vi "Generate Module Definition.vi"(10 "数组":string[][](array[string]), 11 "模块名称":string) -> (3 "模块定义":T1)   [LabVIEW 2018, in "MainInterface.lvlib"]
uses:
  MainInterface.lvlib
  ModuleInterface/ModuleDefinition.ctl
  ModuleInterface/FunctionItem.ctl
  ModuleInterface/ModuleInterface.lvlib
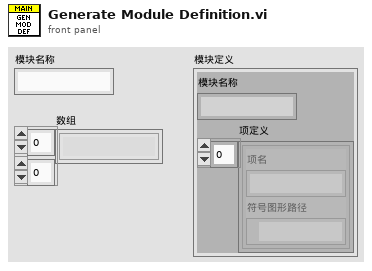
[diagram p1: front panel]
types:
  T1 = typedef "ModuleInterface.lvlib/ModuleDefinition.ctl" = cluster{"模块名称":string, "项定义":T2[]}
  T2 = typedef "ModuleInterface.lvlib/FunctionItem.ctl" = cluster{"项名":string, "符号图形路径":path}
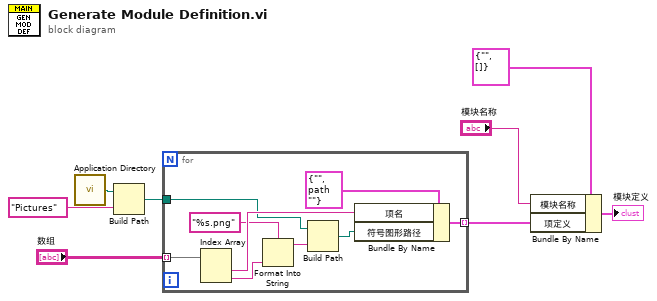
[diagram p0: block diagram]
diagram:
  n1 = call <vilib>:"Application Directory.vi"() -> ("Application Directory"=w2:path)
  n2 = Build Path(base path=w2, name or relative path="Pictures" ("名称或相对路径")) -> (appended path=w1:path)
  n3 = for {
    tunnel: "数组" -> [w16] mode=indexing
    tunnel: w1 -> [w14]
    tunnel: [w10] -> w7 mode=indexing
    n4 = Index Array(array=w16) -> (element #1=w15:string, element #2=w13:string)  [unwired: 2 in]
    n5 = Format Into String(format string="%s.png" ("格式字符串"), w13) -> (resulting string=w11:string)  [unwired: 2 in, 1 out]
    n6 = Build Path(base path=w14, name or relative path=w11) -> (appended path=w9:path)
    n7 = Bundle By Name(cluster=T2 {"项名"="", "符号图形路径"=path ""} ("簇"), "项名"=w15, "符号图形路径"=w9) -> (w10:T2)
  }
  n8 = Bundle By Name(cluster=T1 {"模块名称"="", "项定义"=[]} ("模块定义"), "模块名称"="模块名称", "项定义"=w7) -> (→"模块定义":T1)
